vi "Get Env Var Value.vi"(10 "env var name":string, 11 "default value":string) -> (3 "result":string)   [LabVIEW 2024, in "Sift TDMS Uploader.lvlib" / "Sift TDMS Uploader.lvclass"]
doc: "Reads value from environment variable if it exists otherwise returns default value."
uses:
  Sift TDMS Uploader.lvclass
  <vilib>/Utility/error.llb/Trim Whitespace One-Sided.vi
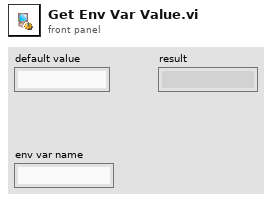
[diagram p1: front panel]
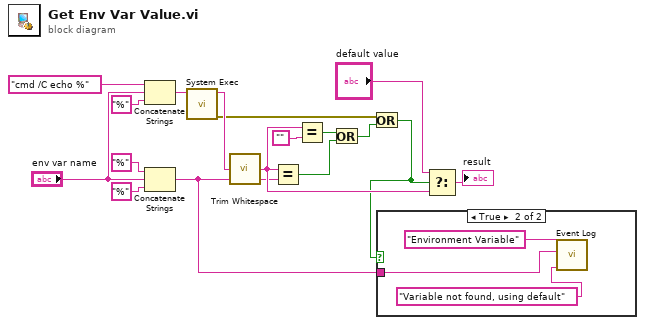
[diagram p0: block diagram]
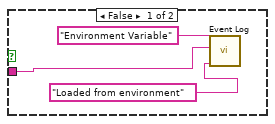
[diagram p2: hidden frame]
diagram:
  n1 = Concatenate Strings("cmd /C echo %", "env var name", "%") -> (w11:string)
  n2 = Concatenate Strings("%", "env var name", "%") -> (w1:string)
  n3 = call <vilib>:"System Exec.vi"("command line"=w11) -> ("error out"=w5:errorcluster, "standard output"=w7:string)  [unwired: 7 in, 2 out]
  n4 = call <vilib>:"Trim Whitespace.vi"("string"=w7) -> ("trimmed string"=w6:string)  [unwired: 1 in]
  n5 = Equal?(x=w6, y=w1) -> (x = y?=w8:bool)
  n6 = Equal?(x=w6, y="") -> (x = y?=w15:bool)
  n7 = Or(x=w15, y=w8) -> (x .or. y?=w4:bool)
  n8 = Or(x=w5, y=w4) -> (x .or. y?=w3:bool)
  n9 = case shown="True" w3 {
    tunnel: w1 -> [w18 w22]
    frame False {
      n10 = call "Event Log.vi"("Message"="Loaded from environment", "Event Type"=w18, "Location"="Environment Variable") -> ()  [unwired: 9 in]
    }
    frame True {
      n11 = call "Event Log.vi"("Message"="Variable not found, using default", "Event Type"=w22, "Location"="Environment Variable") -> ()  [unwired: 9 in]
    }
  }
  n12 = Select(t="default value", s=w3, f=w6) -> (s? t:f=→"result":string)
